vi "Channel Probe_Background Updater.vi"(6 "Subpanels":refnum<vi>[](array[refnum]), 9 "Message Index ref":refnum<vi>, 10 "elements":refnum<vi>, 11 "VI Ref":refnum<vi>) -> ()   [LabVIEW 2019, in "MessengerM.lvlib"]
uses:
  <resource>/Channels/MessengerM/MessengerM.lvlib
  <resource>/Channels/MessengerM/Element.ctl
  <vilib>/ChannelSupport/Channel Message/Channel Message.lvclass
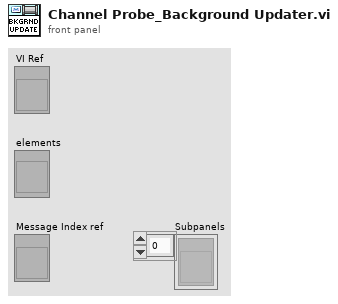
[diagram p1: front panel]
types:
  T1 = typedef "MessengerM.lvlib/Element.ctl" = string
  T2 = enum32{"Bad", "Idle", "Run top level", "Running"}
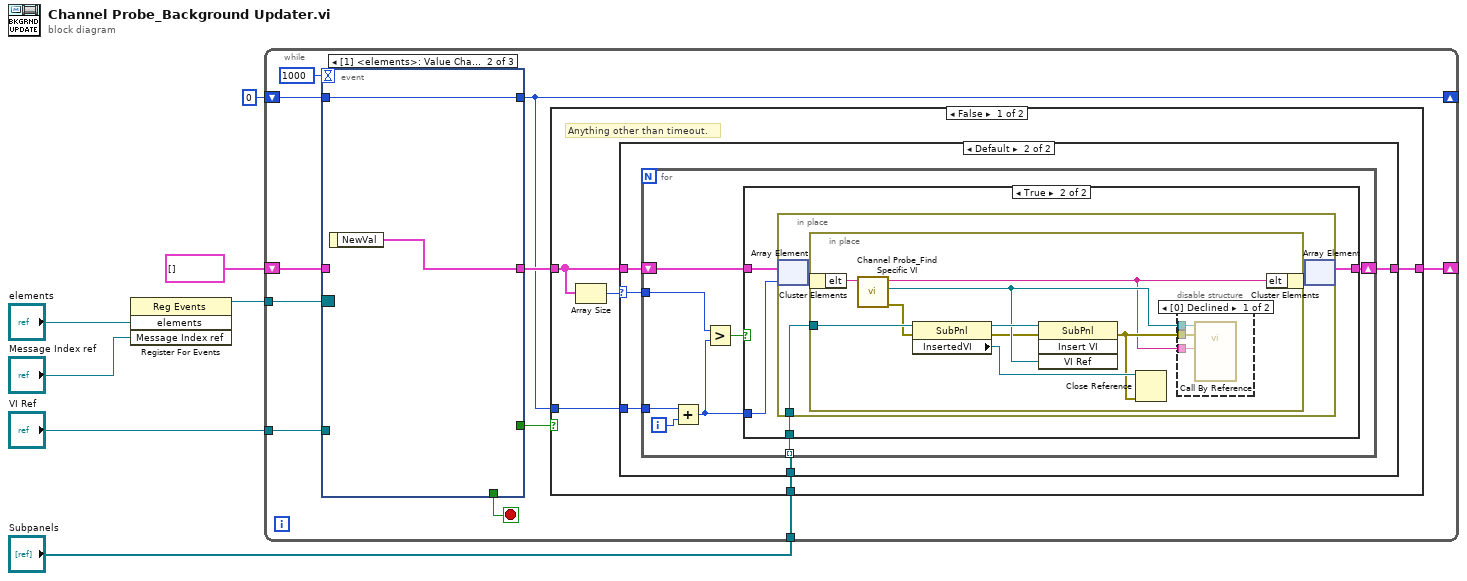
[diagram p0: block diagram]
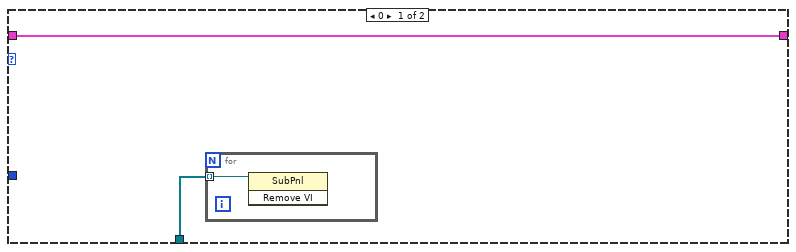
[diagram p2: hidden frame]
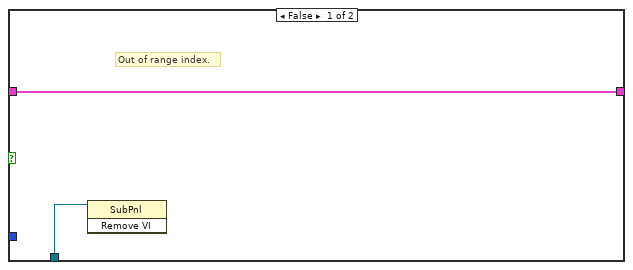
[diagram p3: hidden frame]
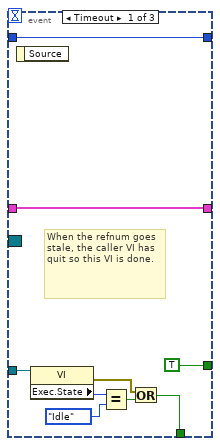
[diagram p6: hidden frame]
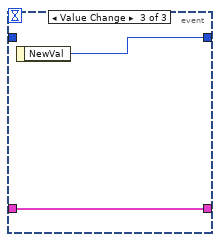
[diagram p7: hidden frame]
diagram:
  n1 = register-events("elements", "Message Index ref") -> (reference out=w5:refnum<event-registration>)  [unwired: 2 in, 1 out]
  n2 = while {
    tunnel: "VI Ref" -> [w17]
    tunnel: w5 -> [w16]
    shift-right: [w12] -> _
    shift-left: cluster{"elt":T1}[] [] ("array") -> [w15]
    shift-right: [w8] -> _
    shift-left: 0 ("NewVal") -> [w14]
    tunnel: "Subpanels" -> [w10]
    stop <- w9 stop-if-true
    n3 = event shown="[1] <elements>: Value Change" {
      selector: w16 -> [_ _ _]
      dyn-events: _ -> [_ _ _]
      timeout: 1000 -> [_ _ _]
      tunnel: w17 -> [w67 _ _]
      tunnel: [w69 w71 w73] -> w11
      tunnel: w15 -> [w69 _ w73]
      tunnel: [w70 w72 w74] -> w8
      tunnel: w14 -> [w70 w72 _]
      tunnel: [TRUE _ _] -> w13
      tunnel: [w62 _ _] -> w9
      event Timeout {
        # "When the refnum goes stale, the caller VI has quit so this VI is done."
        n4 = event-data() -> ()  [unwired: 1 in, 1 out]
        n5 = property class="VI"(reference=w67) -> (error out=w63:errorcluster, "Exec.State"=w66:T2)  [unwired: 1 in, 1 out]
        n6 = Equal?(x=w66, y=T2."Idle") -> (x = y?=w64:bool)
        n7 = Or(x=w63, y=w64) -> (x .or. y?=w62:bool)
      }
      event Value Change {
        n8 = event-data() -> ("NewVal"=w71:cluster{"elt":T1}[])  [unwired: 1 in]
      }
      event Value Change {
        n9 = event-data() -> ("NewVal"=w74:i32)  [unwired: 1 in]
      }
    }
    n10 = case shown="False" w13 {
      tunnel: [w22 w61] -> w12
      tunnel: w11 -> [w21 w61]
      tunnel: w8 -> [w20 _]
      tunnel: w10 -> [w19 _]
      frame False {
        # "Anything other than timeout."
        n11 = Array Size(array=w21) -> (size(s)=w23:i32)
        n12 = case shown="Default" w23 {
          selector: w23 -> [_ w30]
          tunnel: [w25 w29] -> w22
          tunnel: w21 -> [w25 w28]
          tunnel: w20 -> [_ w27]
          tunnel: w19 -> [w24 w31]
          frame 0 {
            n13 = for {
              tunnel: w24 -> [w26] mode=indexing
              n14 = invoke class="SubPnl" method="Remove VI"(reference=w26) -> ()  [unwired: 2 in, 3 out]
            }
          }
          frame Default {
            n15 = for {
              tunnel: w27 -> [w39]
              tunnel: w30 -> [w37]
              tunnel: w31 -> [w35] mode=indexing
              shift-right: [w34] -> w29
              shift-left: w28 -> [w33]
              i -> [w38]
              n16 = Add(x=w39, y=w38) -> (x+y=w32:i32)
              n17 = Greater?(x=w37, y=w32) -> (0:w36:bool)
              n18 = case shown="True" w36 {
                tunnel: w35 -> [w41 w44]
                tunnel: w33 -> [w40 w45]
                tunnel: w32 -> [_ w42]
                tunnel: [w40 w43] -> w34
                frame False {
                  # "Out of range index."
                  n19 = invoke class="SubPnl" method="Remove VI"(reference=w41) -> ()  [unwired: 2 in, 3 out]
                }
                frame True {
                  n20 = in-place {
                    in-place-border: w44 -> [w48]
                    n21 = in-place-array #1(w45, w42) -> (w47:cluster{"elt":T1})
                    n22 = in-place {
                      in-place-border: w48 -> [w56]
                      n23 = in-place-cluster #2(w47) -> ("elt"=w50:T1)
                      n24 = call <resource>:"Channel Probe_Find Specific VI.vi"("element in"=w50) -> ("error out"=w52:errorcluster, "VI Refnum"=w54:refnum<vi>, "element in"=w49:T1)  [unwired: 8 in]
                      n25 = property class="SubPnl"(reference=w56, error in=w52) -> (reference out=w55:refnum<vi>, error out=w51:errorcluster, "InsertedVI"=w57:refnum<vi>)
                      n26 = invoke class="SubPnl" method="Insert VI"(reference=w55, error in=w51, "VI Ref"=w54) -> (error out=w53:errorcluster)  [unwired: 1 in, 3 out]
                      n27 = Close Reference(reference=w57, error in (no error)=w53) -> ()  [unwired: 1 out]
                      n28 = disable-structure shown="[0] Declined" {
                        disable-tunnel: w54 -> [w60 _]
                        disable-tunnel: w49 -> [w59 _]
                        disable-tunnel: w53 -> [w58 _]
                        frame Disabled {
                          n29 = call-by-ref "?"(reference=w60, error in=w58, "Message"=w59) -> ()  [unwired: 11 in, 2 out]
                        }
                        frame Enabled {
                        }
                      }
                      n30 = in-place-cluster #2("elt"=w49) -> (w46:cluster{"elt":T1})
                    }
                    n31 = in-place-array #1(w46) -> (w43:cluster{"elt":T1}[])  [unwired: 1 out]
                  }
                }
              }
            }
          }
        }
      }
      frame True {
      }
    }
  }
